vi "LVClass_WavefrontCorrectorSet dtor.vi"(0 "WavefrontCorrectorSet in":refnum<class "WavefrontCorrectorSet.lvclass">, 11 "error in (no error)":errorcluster) -> (4 "WavefrontCorrectorSet out":refnum<class "WavefrontCorrectorSet.lvclass">, 15 "error out":errorcluster)   [LabVIEW 2020, in "WavefrontCorrectorSet.lvclass"]
doc: "WavefrontCorrectorSet destructor.\n\n--------------------------------------------------------------------------------\n\n<B>wavefrontcorrector_setIn </B> : WavefrontCorrectorSet object.\n<B>wavefrontcorrector_setOut </B> : WavefrontCorrectorSet object.\n<B>ErrorIn </B> : Error\n<B>ErrorOut </B> : Error\n\n--------------------------------------------------------------------------------"
uses:
  WavefrontCorrectorSet.lvclass
  Controls/Wavefront Corrector states - ONE.ctl
  WavefrontCorrectorSet.lvclass/WavefrontCorrectorSet.ctl
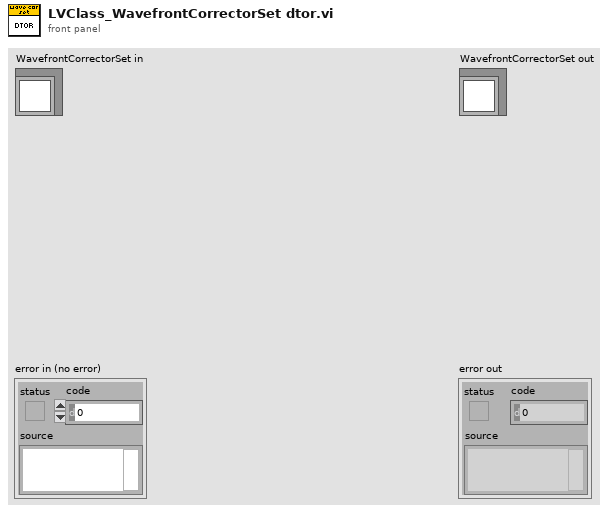
[diagram p1: front panel]
types:
  T1 = typedef "Wavefront Corrector states - ONE.ctl" = cluster{"Max":sgl, "Min":sgl, "Validity":enum16{"valid", "fixed", "invalid"}, "Fixed_Position":sgl}
  T2 = typedef "Handle creation.ctl" = enum16{"By ctor", "By write function"}
  T3 = typedef "ClassID.ctl" = i64
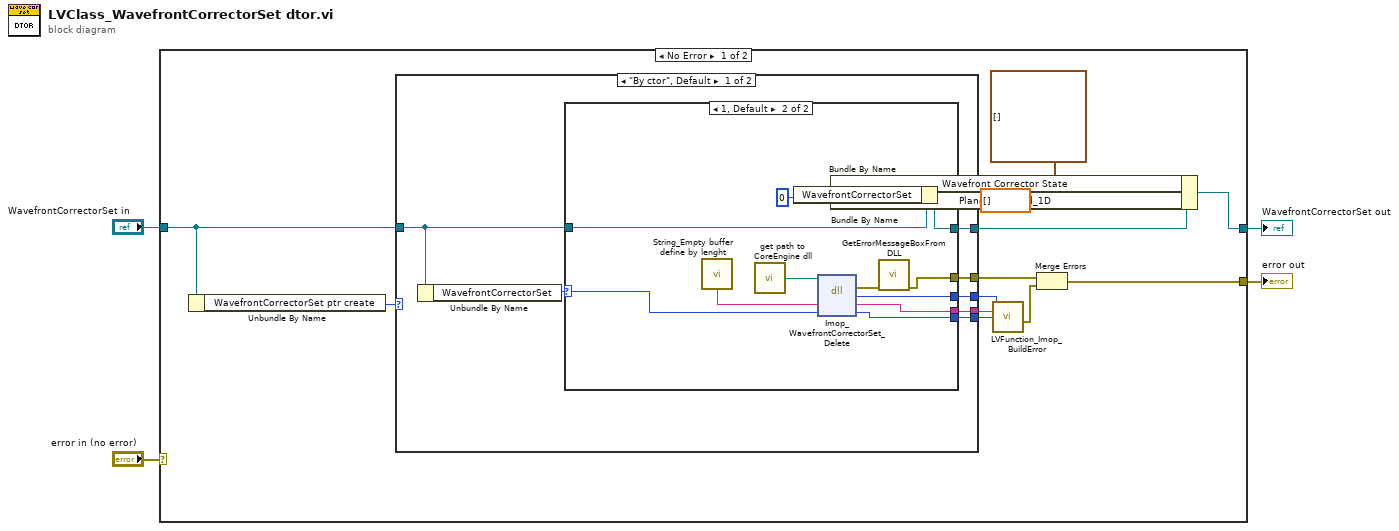
[diagram p0: block diagram]
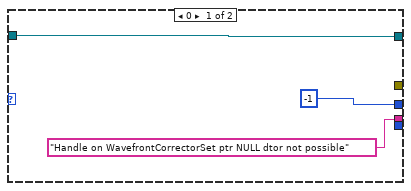
[diagram p2: hidden frame]
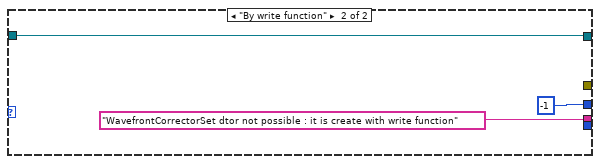
[diagram p3: hidden frame]
diagram:
  n1 = case shown="No Error" "error in (no error)" {
    selector: "error in (no error)" -> [_ w41]
    tunnel: "WavefrontCorrectorSet in" -> [w14 w42]
    tunnel: [w8 w42] -> w2
    tunnel: [w10 w41] -> w1
    frame No Error {
      n2 = Unbundle By Name(w14) -> ("WavefrontCorrectorSet ptr create"=w13:T2)
      n3 = case shown="\"By ctor\", Default" w13 {
        tunnel: [w23 "WavefrontCorrectorSet dtor not possible : it is create with write function" ("message")] -> w16
        tunnel: [w22 -1] -> w15
        tunnel: w14 -> [w20 w38]
        tunnel: [w21 w38] -> w9
        tunnel: [w18 _] -> w12
        tunnel: [w17 _] -> w5
        frame "By ctor", Default {
          n4 = Unbundle By Name(w20) -> ("WavefrontCorrectorSet"=w19:T3)
          n5 = case shown="1, Default" w19 {
            selector: w19 -> [_ w34]
            tunnel: ["Handle on WavefrontCorrectorSet ptr NULL dtor not possible" ("message") w36] -> w23
            tunnel: [-1 w35] -> w22
            tunnel: w20 -> [w24 w30]
            tunnel: [w24 w29] -> w21
            tunnel: [_ w28] -> w18
            tunnel: [_ w27] -> w17
            frame 0 {
            }
            frame 1, Default {
              n6 = call "String_Empty buffer define by lenght.vi"() -> ("Empty buffer"=w37:string)  [unwired: 1 in]
              n7 = call "get path to CoreEngine dll.vi"() -> ("path to wavekit library"=w33:path)  [unwired: 14 in, 1 out]
              n8 = Bundle By Name(cluster=w30, "WavefrontCorrectorSet"=u32 0 ("HasoEgine")) -> (w29:refnum<class "WavefrontCorrectorSet.lvclass">)
              n9 = dll-call lib="D:/soft/HASO_v3/SVN_trunk/ImOpCoreEngine4_LV2011/DLLs/c_interface_vc100.dll" fn="Imop_WavefrontCorrectorSet_Delete"(path in=w33, "message"=w37, "WavefrontCorrectionSet"=w34) -> (error out=w32:errorcluster, "return type"=w35:i32, "message"=w36:string, "WavefrontCorrectionSet"=w27:i64)  [unwired: 2 in, 1 out]
              n10 = call "GetErrorMessageBoxFromDLL.vi"("error IN"=w32) -> ("error OUT"=w28:errorcluster)  [unwired: 10 in]
            }
          }
        }
        frame "By write function" {
        }
      }
      n11 = Bundle By Name(cluster=w9, "Wavefront Corrector State"=T1[] [], "PlaneCommand_1D"=sgl[] []) -> (w8:refnum<class "WavefrontCorrectorSet.lvclass">)
      n12 = call "LVFunction_Imop_BuildError.vi"("code"=w15, "String to Prepend to source (\"\")"=w16, "Adresse"=w5) -> ("error out"=w11:errorcluster)  [unwired: 12 in]
      n13 = Merge Errors(w12, w11) -> (w10:errorcluster)
    }
    frame Error {
    }
  }
  "error out" <- w1
  "WavefrontCorrectorSet out" <- w2
